vi "RSZVB Set DC Value.vi"(8 "error in (no error)":errorcluster {"code" format="%.0x"}, 9 "DC Value (0.0)":dbl format="%^.3e", 10 "Channel (Trace) (1)":i32=1, 11 "VISA session":refnum<visa-resource-name>) -> (0 "error out":errorcluster {"code" format="%.0x"}, 3 "dup VISA session":refnum<visa-resource-name>)   [LabVIEW 2011]
doc: "This VI sets the DC value for low pass transforms. The VI is enabled only if the sweep points are on a harmonic grid (to be set explicitly or using CALCulate<Ch/Tr>:TRANsform:TIME:LPASs).\n\nRemote-control command(s):\nCALCulate<Ch/Tr>:TRANsform:TIME:LPASs:DCSParam"
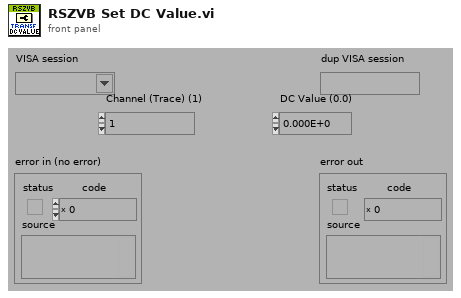
[diagram p1: front panel]
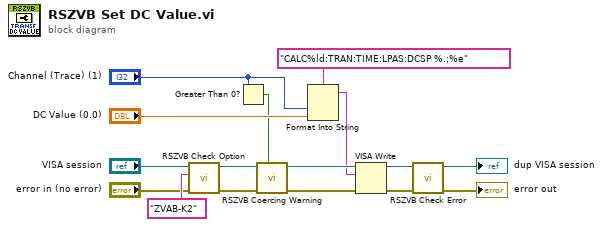
[diagram p0: block diagram]
diagram:
  n1 = call "RSZVB Check Option.vi"("error in (no error)"="error in (no error)", "Options"="ZVAB-K2", "VISA session"="VISA session") -> ("error out"=w8:errorcluster, "dup VISA session"=w9:refnum<visa-resource-name>)  [unwired: 7 in]
  n2 = Greater Than 0?(x="Channel (Trace) (1)") -> (x > 0?=w1:bool)
  n3 = call "RSZVB Coercing Warning.vi"("In Range?"=w1, "error in (no error)"=w8, "VISA session"=w9) -> ("error out"=w14:errorcluster, "dup VISA session"=w15:refnum<visa-resource-name>)  [unwired: 7 in]
  n4 = Format Into String(format string="CALC%ld:TRAN:TIME:LPAS:DCSP %.;%e", "Channel (Trace) (1)", "DC Value (0.0)") -> (resulting string=w11:string)  [unwired: 2 in, 1 out]
  n5 = VISA Write(VISA resource name=w15, write buffer=w11, error in (no error)=w14) -> (VISA resource name out=w12:refnum<visa-resource-name>, error out=w13:errorcluster)  [unwired: 1 out]
  n6 = call "RSZVB Check Error.vi"("error in (no error)"=w13, "VISA session"=w12) -> ("error out"=→"error out":errorcluster, "dup VISA session"=→"dup VISA session":refnum<visa-resource-name>)  [unwired: 8 in]
